vi "Graph.vi"(4 "Resistances In":dbl[][](array[numeric]), 6 "Array in":T2[](array[typedef]) {"MassFlow" format="%.2f"; "Setpoint" format="%.2f"}, 8 "error in (no error)":errorcluster, 9 "T  (ºC)":dbl format="%.2g", 10 "RH  (%)":dbl format="%.2g", 11 "Ethanol (%)":dbl format="%.3g") -> (0 "error out":errorcluster, 3 "Cluster":T1)   [LabVIEW 2019, in "DAQ.lvclass"]
uses:
  DAQ.lvclass
  typeDefs/MFCOut.ctl
  typeDefs/Graph.ctl
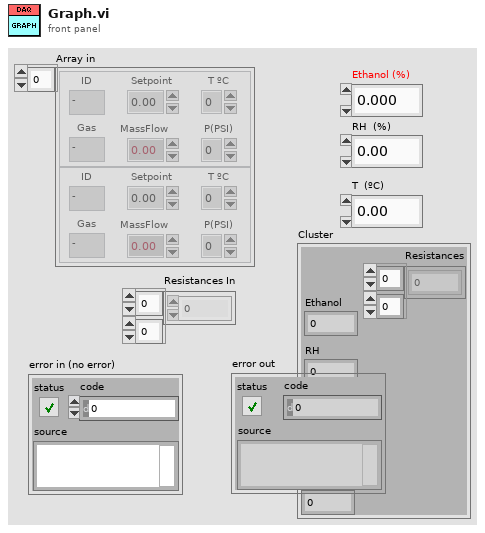
[diagram p1: front panel]
types:
  T1 = typedef "Graph.ctl" = cluster{"Ethanol":dbl, "RH":dbl, "Temp":dbl, "MFC A":dbl, "MFC B":dbl, "Resistances":dbl[][]}
  T2 = typedef "MFCOut.ctl" = cluster{"Gas":string, "Setpoint":dbl, "MassFlow":dbl, "T ºC":dbl, "P(PSI)":dbl, "ID":string}
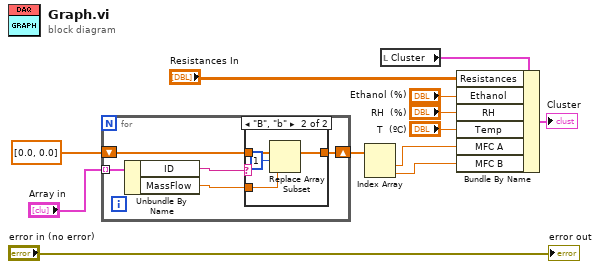
[diagram p0: block diagram]
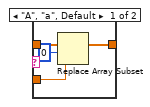
[diagram p2: hidden frame]
diagram:
  n1 = for {
    tunnel: "Array in" -> [w17] mode=indexing
    shift-right: [w14] -> w11
    shift-left: dbl[] [0.0, 0.0] -> [w15]
    n2 = Unbundle By Name(w17) -> ("ID"=w16:string, "MassFlow"=w13:dbl)
    n3 = case shown="\"B\", \"b\"" w16 {
      tunnel: [w21 w25] -> w14
      tunnel: w15 -> [w20 w24]
      tunnel: w13 -> [w19 w23]
      frame "A", "a", Default {
        n4 = Replace Array Subset(array=w20, new element=w19, index=0) -> (w21:dbl[])
      }
      frame "B", "b" {
        n5 = Replace Array Subset(array=w24, new element=w23, index=1) -> (w25:dbl[])
      }
    }
  }
  n6 = Index Array(array=w11) -> (element #1=w2:dbl, element #2=w12:dbl)  [unwired: 2 in]
  n7 = local read "Cluster"() -> (w3:T1)
  n8 = Bundle By Name(cluster=w3, "Resistances"="Resistances In", "Ethanol"="Ethanol (%)", "RH"="RH  (%)", "Temp"="T  (ºC)", "MFC A"=w2, "MFC B"=w12) -> (→"Cluster":T1)
  "error out" <- "error in (no error)"
